vi "Stop FV Pump.vi"(8 "error in (no error)":errorcluster) -> (0 "error out":errorcluster)   [LabVIEW 2015]
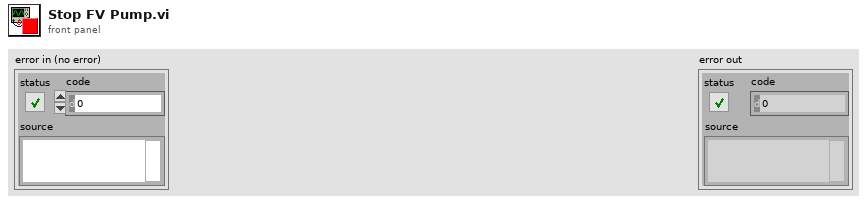
[diagram p1: front panel]
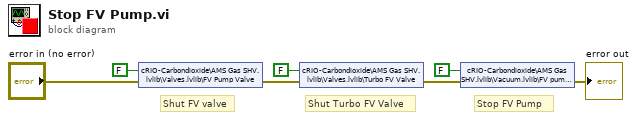
[diagram p0: block diagram]
diagram:
  # "Stop FV Pump"
  # "Shut Turbo FV Valve"
  # "Shut FV valve"
  n1 = shared-variable "cRIO-Carbondioxide\\AMS Gas SHV.lvlib\\Valves.lvlib\\FV Pump Valve"(FALSE ("FV pump valve"), error in="error in (no error)") -> (error out=w2:errorcluster)
  n2 = shared-variable "cRIO-Carbondioxide\\AMS Gas SHV.lvlib\\Valves.lvlib\\Turbo FV Valve"(FALSE ("FV pump valve"), error in=w2) -> (error out=w1:errorcluster)
  n3 = shared-variable "cRIO-Carbondioxide\\AMS Gas SHV.lvlib\\Vacuum.lvlib\\FV pump ON"(FALSE ("FV pump valve"), error in=w1) -> (error out=→"error out":errorcluster)
